vi "Close.vi"(8 "error in (no error)":errorcluster, 11 "KUKA youBot arm motor in":refnum<class "NI_Robotics_KUKA youBot Arm Motor.lvclass">) -> (0 "error out":errorcluster)   [LabVIEW 2017, in "NI_Robotics_KUKA youBot Host.lvlib" / "NI_Robotics_KUKA youBot Arm Motor.lvclass"]
uses:
  <vilib>/robotics/KUKA youBot/Motor/Arm Motor/NI_Robotics_KUKA youBot Arm Motor.lvclass
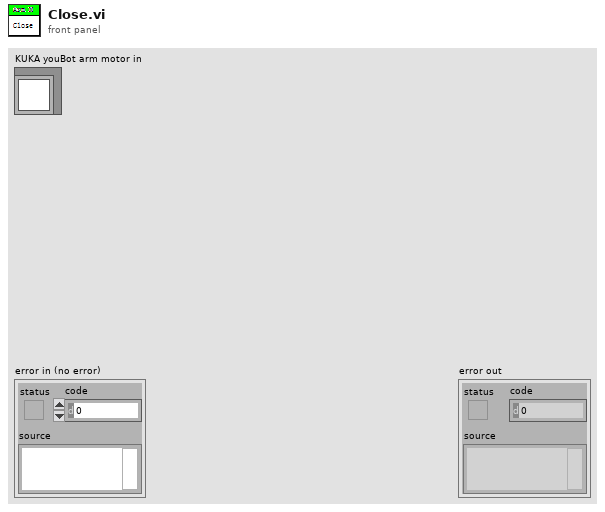
[diagram p1: front panel]
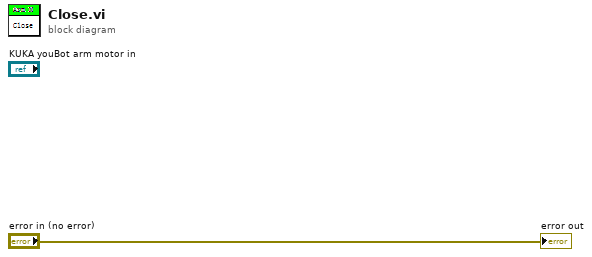
[diagram p0: block diagram]
diagram:
  "error out" <- "error in (no error)"
